vi "Write Behavior.vi"(10 "match behavior":T1, 11 "Filter in":refnum<class "Filter.lvclass">) -> (3 "Filter out":refnum<class "Filter.lvclass">)   [LabVIEW 2018, in "Logging.lvlib" / "Filter.lvclass"]
uses:
  Filter.lvclass
  Match Behavior.ctl
  Filter.lvclass/Filter.ctl
  Logging.lvlib
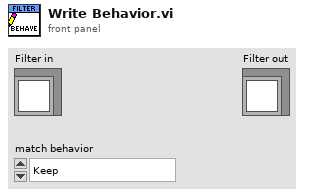
[diagram p1: front panel]
types:
  T1 = typedef "Logging.lvlib/Match Behavior.ctl" = enum16{"Keep", "Discard"}
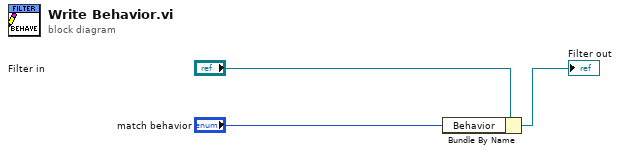
[diagram p0: block diagram]
diagram:
  n1 = Bundle By Name(cluster="Filter in", "Behavior"="match behavior") -> (→"Filter out":refnum<class "Filter.lvclass">)
